vi "Read Single.vi"(0 "RS232 Port In":refnum<visa-resource-name>="COM12", 1 "Sensor Address In":string="0", 4 "Measurement Type In (Normal)":i32(ring) items=["Normal", "Concurrent", "Continuous"], 5 "CRC (False)":bool, 6 "Parameter In (0)":i32(ring) items=["0", "1", "2", "3", "4", "5", "6", "7", "8", "9"], 7 "Error In (No Error)":errorcluster, 10 "Initialize/close":bool) -> (20 "RS232 Port Out":refnum<visa-resource-name>="COM1", 21 "Sensor Address Out":string="a" caption="sensor address out", 22 "Measurements Out":dbl[](array[numeric]), 23 "Number of Measurements Out":i32, 24 "Measurement Type Out":i32(ring) items=["Normal", "Concurrent", "Continuous"], 25 "CRC Out":bool, 26 "Parameter Out":i32(ring) items=["0", "1", "2", "3", "4", "5", "6", "7", "8", "9"], 27 "Error Out":errorcluster)   [LabVIEW 2016, in "SDI-12.lvlib"]
doc: "Creates and sends a single measurement command toa sensor, and reads the measurement response(s). \n\nThe amount of data measured depends on settings of each sensor, and these settings are not ecompassed by the SDI-12 protocol.\n\nFor Normal/Concurrent Measurement Types, Read Single calls:\n1. Initiate Measurement.\n2. Wait.\n3. Fetch.\n\nFor Continuous Measurements, Read Single calls:\n1. Fetch.\n\nVisit http://www.sdi-12.org/ for more information on the SDI-12 protocol."
uses:
  SDI-12.lvlib
panel:
  out "elapsed time":dbl
  out "Max Acquisition Time (sec)":i32
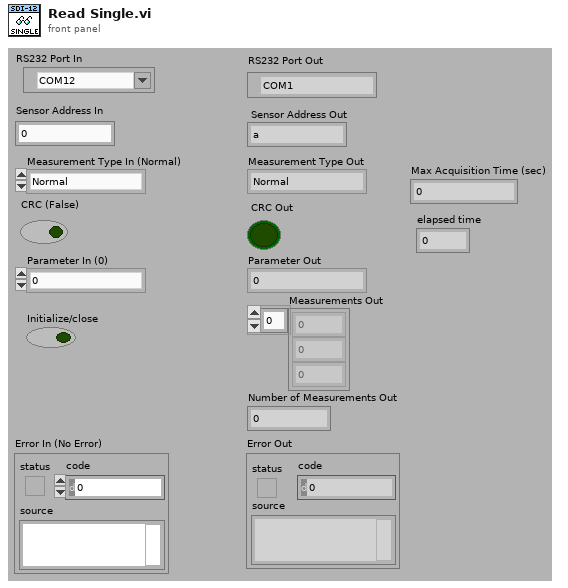
[diagram p1: front panel]
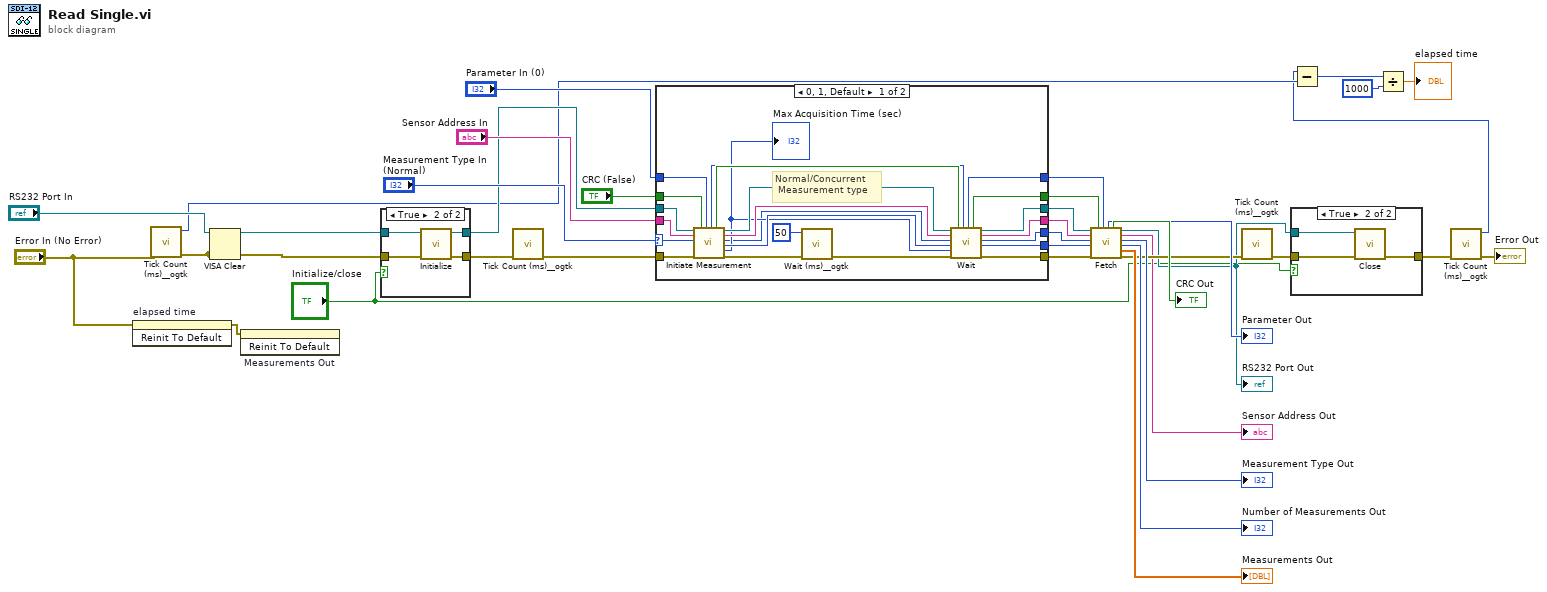
[diagram p0: block diagram]
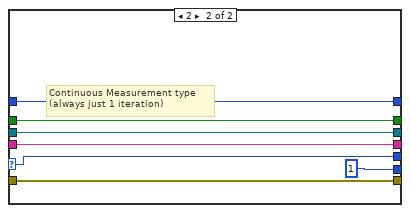
[diagram p4: hidden frame]
diagram:
  n1 = invoke on="elapsed time" class="DigNum (strict)" method="Reinit To Default"(error in="Error In (No Error)") -> (error out=w1:errorcluster)  [unwired: 2 in, 2 out]
  n2 = call <userlib>:"Tick Count (ms)__ogtk.vi"("error in (no error)"="Error In (No Error)") -> ("error out"=w3:errorcluster, "millisecond timer value"=w6:u32)  [unwired: 9 in]
  n3 = VISA Clear(VISA resource name="RS232 Port In", error in (no error)=w3) -> (VISA resource name out=w4:refnum<visa-resource-name>)  [unwired: 1 out]
  n4 = invoke on="Measurements Out" class="Arr (strict)" method="Reinit To Default"(error in=w1) -> ()  [unwired: 2 in, 3 out]
  n5 = case shown="True" "Initialize/close" {
    tunnel: w3 -> [w38 w42]
    tunnel: w4 -> [w37 w41]
    tunnel: [w38 w40] -> w14
    tunnel: [w37 w39] -> w13
    frame False {
    }
    frame True {
      n6 = call "Initialize.vi"("Error In (No Error)"=w42, "RS232 Port In"=w41) -> ("Error Out"=w40:errorcluster, "RS232 Port Out"=w39:refnum<visa-resource-name>)  [unwired: 8 in]
    }
  }
  n7 = call <userlib>:"Tick Count (ms)__ogtk.vi"("error in (no error)"=w14) -> ("error out"=w18:errorcluster)  [unwired: 9 in, 1 out]
  n8 = case shown="0, 1, Default" "Measurement Type In (Normal)" {
    selector: "Measurement Type In (Normal)" -> [w45 w67]
    tunnel: w18 -> [w65 w70]
    tunnel: "CRC (False)" -> [w64 w72]
    tunnel: "Parameter In (0)" -> [w63 w71]
    tunnel: [w58 w67] -> w19
    tunnel: [w57 1 ("Number of Measurements Out")] -> w34
    tunnel: [w56 w70] -> w33
    tunnel: [w53 w71] -> w32
    tunnel: [w52 w72] -> w31
    tunnel: w13 -> [w46 w69]
    tunnel: [w49 w69] -> w22
    tunnel: [w48 w68] -> w21
    tunnel: "Sensor Address In" -> [w47 w68]
    frame 0, 1, Default {
      # "Normal/Concurrent\n Measurement type"
      n9 = call "Initiate Measurement.vi"("RS232 Port In"=w46, "Sensor Address In"=w47, "Measurement Type In (Normal)"=w45, "Error In (No Error)"=w65, "CRC In (False)"=w64, "Parameter In (0)"=w63) -> ("Parameter Out"=w54:i32, "CRC Out"=w55:bool, "RS232 Port Out"=w61:refnum<visa-resource-name>, "Sensor Address Out"=w60:string, "Measurement Type Out"=w50:i32, "Number of Measurements"=w59:i32, "Max Acquisition Time (sec)"=w51:i32, "Error Out"=w62:errorcluster)  [unwired: 6 in]
      "Max Acquisition Time (sec)" <- w51
      n10 = call <userlib>:"Wait (ms)__ogtk.vi"("error in (no error)"=w62, "milliseconds to wait"=u32 50) -> ("error out"=w44:errorcluster)  [unwired: 8 in, 1 out]
      n11 = call "Wait.vi"("RS232 Port In"=w61, "Sensor Address In"=w60, "Measurement Type In (Normal)"=w50, "Number of Measurements In (1)"=w59, "Max Acquisition Time (0 sec)"=w51, "Error In (No Error)"=w44, "CRC (False)"=w55, "Parameter In (0)"=w54) -> ("Parameter Out"=w53:i32, "CRC Out"=w52:bool, "RS232 Port Out"=w49:refnum<visa-resource-name>, "Sensor Address Out"=w48:string, "Measurement Type Out"=w58:i32, "Number of Measurements Out"=w57:i32, "Error Out"=w56:errorcluster)  [unwired: 5 in]
    }
    frame 2 {
      # "Continuous Measurement type\n(always just 1 iteration)"
    }
  }
  n12 = call "Fetch.vi"("RS232 Port In"=w22, "Sensor Address In"=w21, "Measurement Type In (Normal)"=w19, "Number of Measurements In (1)"=w34, "Error In (No Error)"=w33, "CRC (False)"=w31, "Parameter In (0)"=w32) -> ("Parameter Out"=→"Parameter Out":i32, "CRC Out"=→"CRC Out":bool, "RS232 Port Out"=w9:refnum<visa-resource-name>, "Sensor Address Out"=→"Sensor Address Out":string, "Measurement Type Out"=→"Measurement Type Out":i32, "Number of Measurements Out"=→"Number of Measurements Out":i32, "Measurements Out"=→"Measurements Out":dbl[], "Error Out"=w24:errorcluster)  [unwired: 5 in]
  "RS232 Port Out" <- w9
  n13 = call <userlib>:"Tick Count (ms)__ogtk.vi"("error in (no error)"=w24) -> ("error out"=w11:errorcluster)  [unwired: 9 in, 1 out]
  n14 = case shown="True" "Initialize/close" {
    tunnel: [w73 w76] -> w10
    tunnel: w11 -> [w73 w75]
    tunnel: w9 -> [_ w74]
    frame False {
    }
    frame True {
      n15 = call "Close.vi"("Error In (No Error)"=w75, "RS232 Port In"=w74) -> ("Error Out"=w76:errorcluster)  [unwired: 9 in]
    }
  }
  n16 = call <userlib>:"Tick Count (ms)__ogtk.vi"("error in (no error)"=w10) -> ("error out"=→"Error Out":errorcluster, "millisecond timer value"=w5:u32)  [unwired: 9 in]
  n17 = Subtract(x=w5, y=w6) -> (x-y=w17:u32)
  n18 = Divide(x=w17, y=u32 1000) -> (x/y=→"elapsed time":dbl)
